vi "4-7.vi"() -> ()   [LabVIEW 2017]
panel:
  out "随机的数":i16
  out "循环次数":dbl
  in  "猜测的数":i16
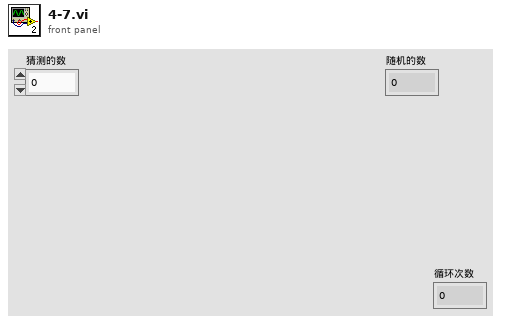
[diagram p1: front panel]
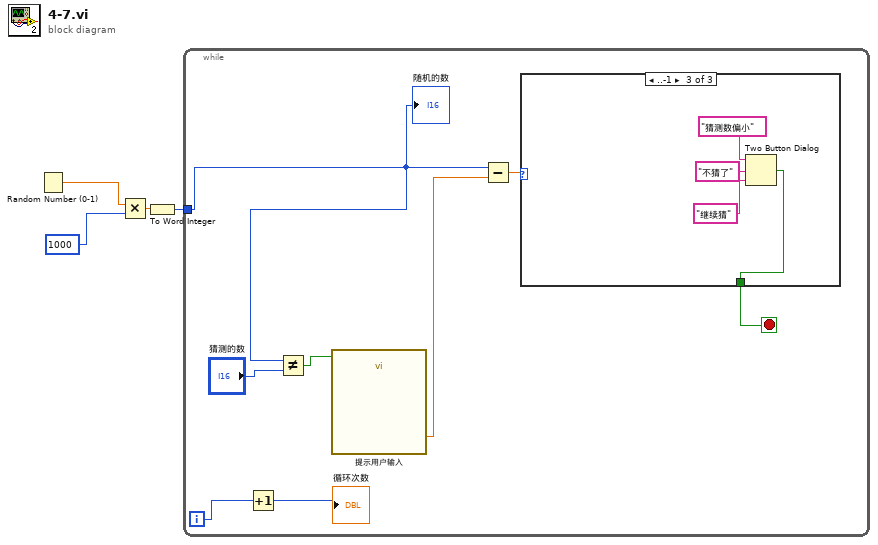
[diagram p0: block diagram]
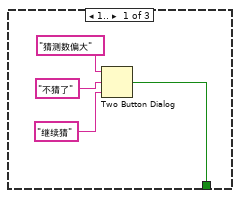
[diagram p2: hidden frame]
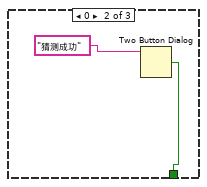
[diagram p3: hidden frame]
diagram:
  n1 = Random Number (0-1)() -> (number: 0 to 1=w4:dbl)
  n2 = Multiply(x=w4, y=1000) -> (x*y=w3:dbl)
  n3 = To Word Integer(number=w3) -> (16bit integer=w1:i16)
  n4 = while {
    tunnel: w1 -> [w5]
    i -> [w12]
    stop <- w6 stop-if-true
    n5 = Increment(x=w12) -> (x+1=→"循环次数":i32)
    n6 = Not Equal?(x=w5, y="猜测的数") -> (x != y?=w9:bool)
    n7 = call "提示用户输入"("Enable"=w9) -> ("请在1—1000猜"=w7:dbl)  [unwired: 16 in, 2 out]
    n8 = Subtract(x=w5, y=w7) -> (x-y=w10:dbl)
    n9 = case shown="..-1" w10 {
      tunnel: [w13 w17 w19] -> w6
      frame 1.. {
        n10 = Two Button Dialog(message="猜测数偏大", 1:"继续猜", 2:"不猜了") -> (T button?=w13:bool)
      }
      frame 0 {
        n11 = Two Button Dialog(message="猜测成功") -> (T button?=w17:bool)  [unwired: 2 in]
      }
      frame ..-1 {
        n12 = Two Button Dialog(message="猜测数偏小", 1:"继续猜", 2:"不猜了") -> (T button?=w19:bool)
      }
    }
    "随机的数" <- w5
  }
